vi "Should Show Tree Edit Control.vi"(11 "UI Data in":refnum<class "Settings UI.lvclass">) -> (1 "Data Type":T1 items=["Tree Parent"=-1, "Numeric"=0, "String"=1, "Boolean"=2, "Enum"=3], 2 "Show Tree Edit Control":bool, 3 "UI Data out":refnum<class "Settings UI.lvclass">)   [LabVIEW 2020, in "Output Sequencer.lvlib" / "Settings UI.lvclass"]
uses:
  Settings UI.lvclass
  Types/Data Type.ctl
  Settings UI.lvclass/Settings UI.ctl
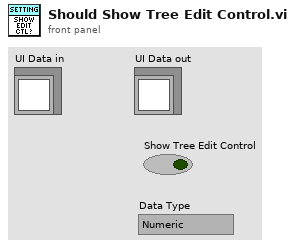
[diagram p1: front panel]
types:
  T1 = typedef "Output Sequencer.lvlib/Settings UI.lvclass/Data Type.ctl" = i16
  T2 = typedef "Output Sequencer.lvlib/Settings UI.lvclass/Tree Item Settings.ctl" = cluster{"Tree Label":string, "Indent Level":i32, "Data Type":T1, "Numeric Range":cluster{"Min":dbl, "Max":dbl, "Inc":dbl}, "Allowed Values":string[], "Default Value":string, "Description":string}
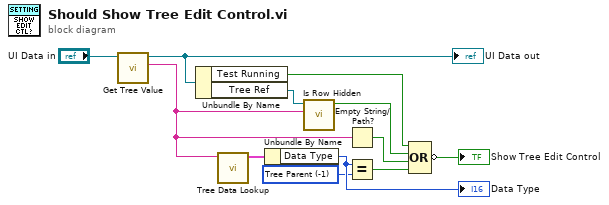
[diagram p0: block diagram]
diagram:
  w7 = T1 -1 items=["Tree Parent"=-1, "Numeric"=0, "String"=1, "Boolean"=2, "Enum"=3, "Command"=4, "Numeric Min/Max"=5] ("Data Type")
  n1 = call "Get Tree Value.vi"("UI Data in"="UI Data in") -> ("Value"=w4:string, "UI Data out"=w11:refnum<class "Settings UI.lvclass">)  [unwired: 9 in]
  "UI Data out" <- w11
  n2 = Unbundle By Name(w11) -> ("Test Running"=w1:bool, "Tree Ref"=w3:refnum<vi>)
  n3 = call "Tree Data Lookup.vi"("Tag in"=w4) -> ("Tree Data"=w8:T2)  [unwired: 5 in, 5 out]
  n4 = Unbundle By Name(w8) -> ("Data Type"=w9:T1)
  "Data Type" <- w9
  n5 = call "Is Row Hidden.vi"("Tag"=w4, "TreeControl in"=w3) -> ("Hidden"=w2:bool)  [unwired: 9 in]
  n6 = Empty String/Path?(string/path=w4) -> (empty?=w5:bool)
  n7 = Equal?(x=w9, y=w7) -> (x = y?=w6:bool)
  n8 = Compound Arithmetic op=OR(w1, w2, w5, w6) -> (invert →"Show Tree Edit Control":bool)
